vi "TCP_READ.vi"(0 "connection ID":refnum<k5>, 1 "error in (no error)":errorcluster) -> (2 "data":string, 3 "connection ID out":refnum<k5>, 4 "error out":errorcluster)   [LabVIEW 2023]
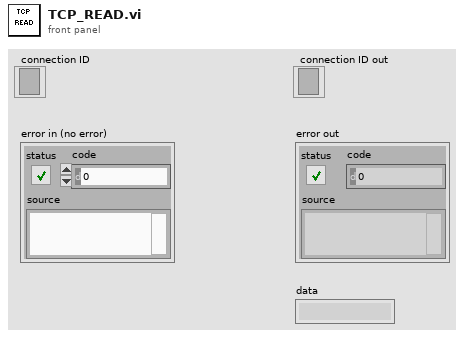
[diagram p1: front panel]
types:
  T1 = enum16{"Standard", "Buffered", "CRLF", "Immediate"}
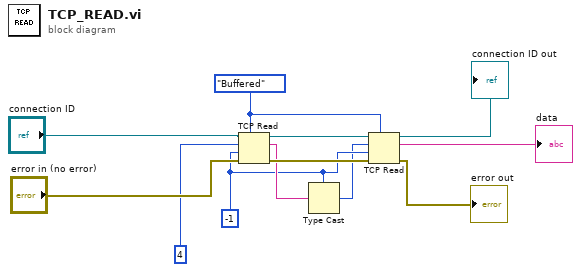
[diagram p0: block diagram]
diagram:
  w4 = T1."Buffered" ("mode (standard)")
  w7 = -1 ("timeout ms (25000)")
  n1 = TCP Read(connection ID="connection ID", bytes to read=4, error in (no error)="error in (no error)", 7:w4, 9:w7) -> (connection ID out=w5:refnum<k5>, data out=w8:string, error out=w9:errorcluster)
  n2 = Type Cast(type=w7, x=w8) -> (*(type *) &x=w6:i32)
  n3 = TCP Read(connection ID=w5, bytes to read=w6, error in (no error)=w9, 7:w4, 9:w7) -> (connection ID out=→"connection ID out":refnum<k5>, data out=→"data":string, error out=→"error out":errorcluster)
